vi "Top-Level.vi"() -> ()   [LabVIEW 2011]
uses:
  <vilib>/Platform/TimedLoop/XDataNode/timing_clust.ctl
  <vilib>/Platform/TimedLoop/XDataNode/nitl_modes.ctl
  <vilib>/Platform/TimedLoop/XDataNode/wakeup.ctl
  <vilib>/rvi/eio/common/nirviEmuTemplateMethod_errors.vi
  <vilib>/eio/EIONode/EIONode.xnode
  <vilib>/Platform/TimedLoop/XDataNode/XDataNode.xnode
  <vilib>/Platform/TimedLoop/XDataNode/XDNodeRunTimeDep.lvlib
panel:
  in  "manual steering":bool
  out "Velocity counts":u32
  in  "Enable AI15":bool
  out "AI15":u16 format="%04d"
  in  "Enable AI14":bool
  out "AI14":u16 format="%04d"
  in  "Enable AI13":bool
  out "AI13":u16 format="%04d"
  in  "Enable AI12":bool
  out "AI12":u16 format="%04d"
  in  "Enable AI11":bool
  out "AI11":u16 format="%04d"
  in  "Enable AI10":bool
  out "AI10":u16 format="%04d"
  in  "Enable AI9":bool
  out "AI9":u16 format="%04d"
  in  "Enable AI8":bool
  out "AI8":u16 format="%04d"
  in  "Enable AI7":bool
  out "AI7":u16 format="%04d"
  in  "Enable AI6":bool
  out "AI6":u16 format="%04d"
  in  "Enable AI5":bool
  out "AI5":u16 format="%04d"
  in  "Enable AI4":bool
  out "AI4":u16 format="%04d"
  in  "Enable AI3":bool
  out "AI3":u16 format="%04d"
  in  "Enable AI2":bool
  out "AI2":u16 format="%04d"
  in  "Enable AI1":bool=TRUE
  out "AI1":u16 format="%04d"
  in  "Enable AI0":bool=TRUE
  out "AI0":u16 format="%04d"
  in  "ADC Run":bool=TRUE
  out "ADC Channel List":u16 format="%016b"
  in  "ADC Reset":bool
  out "Steering ON 1e-7s":u32
  out "Go Duty":u8
  out "Go Frequency":u16
  out "microblaze\\xps_gpio_0_GPIO_IO_O_pin 2":i32
  in  "manual throttle":bool
  out "Brake":bool
  out "Reverse":bool
  out "Enable":bool
  in  "uBlaze Reset":bool
  out "PWM0 period (cycles)":u32=400000
  out "PWM0 duty (cycles)":u32=80000
  in  "Clock Frequency (Hz)":u32=40000000
  out "PWM1 period(cycles)":u32=400000
  out "PWM1 duty (cycles)":u32=80000
  in  "PWM0 frequency (Hz)":u16
  in  "PWM0 duty (100*%)":u16
  in  "PWM1 frequency (Hz)":u16
  in  "PWM1 duty (100*%)":u16
  out "Steering period (cycles)":u32=400000
  out "Steering duty (cycles)":u32=80000
  out "GO period (cycles)":u32=400000
  out "GO duty (cycles)":u32=80000
  in  "Steering frequency (Hz)":u16=50
  in  "Steering ON 1e-7s":u32=8
  in  "GO frequency (Hz)":u16=1000
  in  "GO duty (100*%)":u16
  # "ADC"
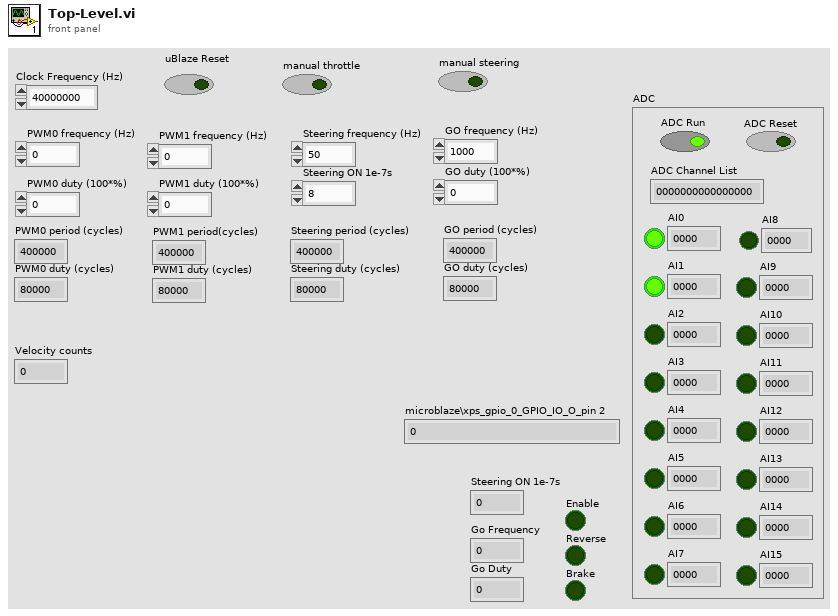
[diagram p1: front panel]
types:
  T1 = typedef "XDNodeRunTimeDep.lvlib/timing_clust.ctl" = cluster{"Expected End [f-1]":u64, "Actual End [f-1]":u64, "Finished Late? [f-1]":bool, "Expected End [i-1]":u64, "Actual End [i-1]":u64, "Finished Late? [i-1]":bool, "Expected Start [i]":u64, "Actual Start [i]":u64, "Expected Start [f]":u64, "Actual Start [f]":u64, "Source Name":string, "Structure Name":string, "Period":i64, "Deadline":i64, "Offset":i64, "Start":i64, "Priority":i32, "Timeout":i32, "Mode":T2, "Wakeup Reason":T3, "Error":errorcluster, "Source Type":string, "Secondary Source Type":string, "Global End Time":u64, "Global Start Time":u64, "Frame Duration":u64, "Iteration Duration":u64, "Assigned CPU":i32, "I/O Scan Engine Mode":u32}
  T2 = typedef "XDNodeRunTimeDep.lvlib/nitl_modes.ctl" = enum32{"No Change", "Process missed periods, maintain original phase", "Discard missed periods, maintain original phase", "Process missed periods, ignore original phase", "Discard missed periods, ignore original phase"}
  T3 = typedef "XDNodeRunTimeDep.lvlib/wakeup.ctl" = enum32{"Normal", "Aborted", "Asynchronous wakeup", "Timing source error", "Timed loop error", "Timeout"}
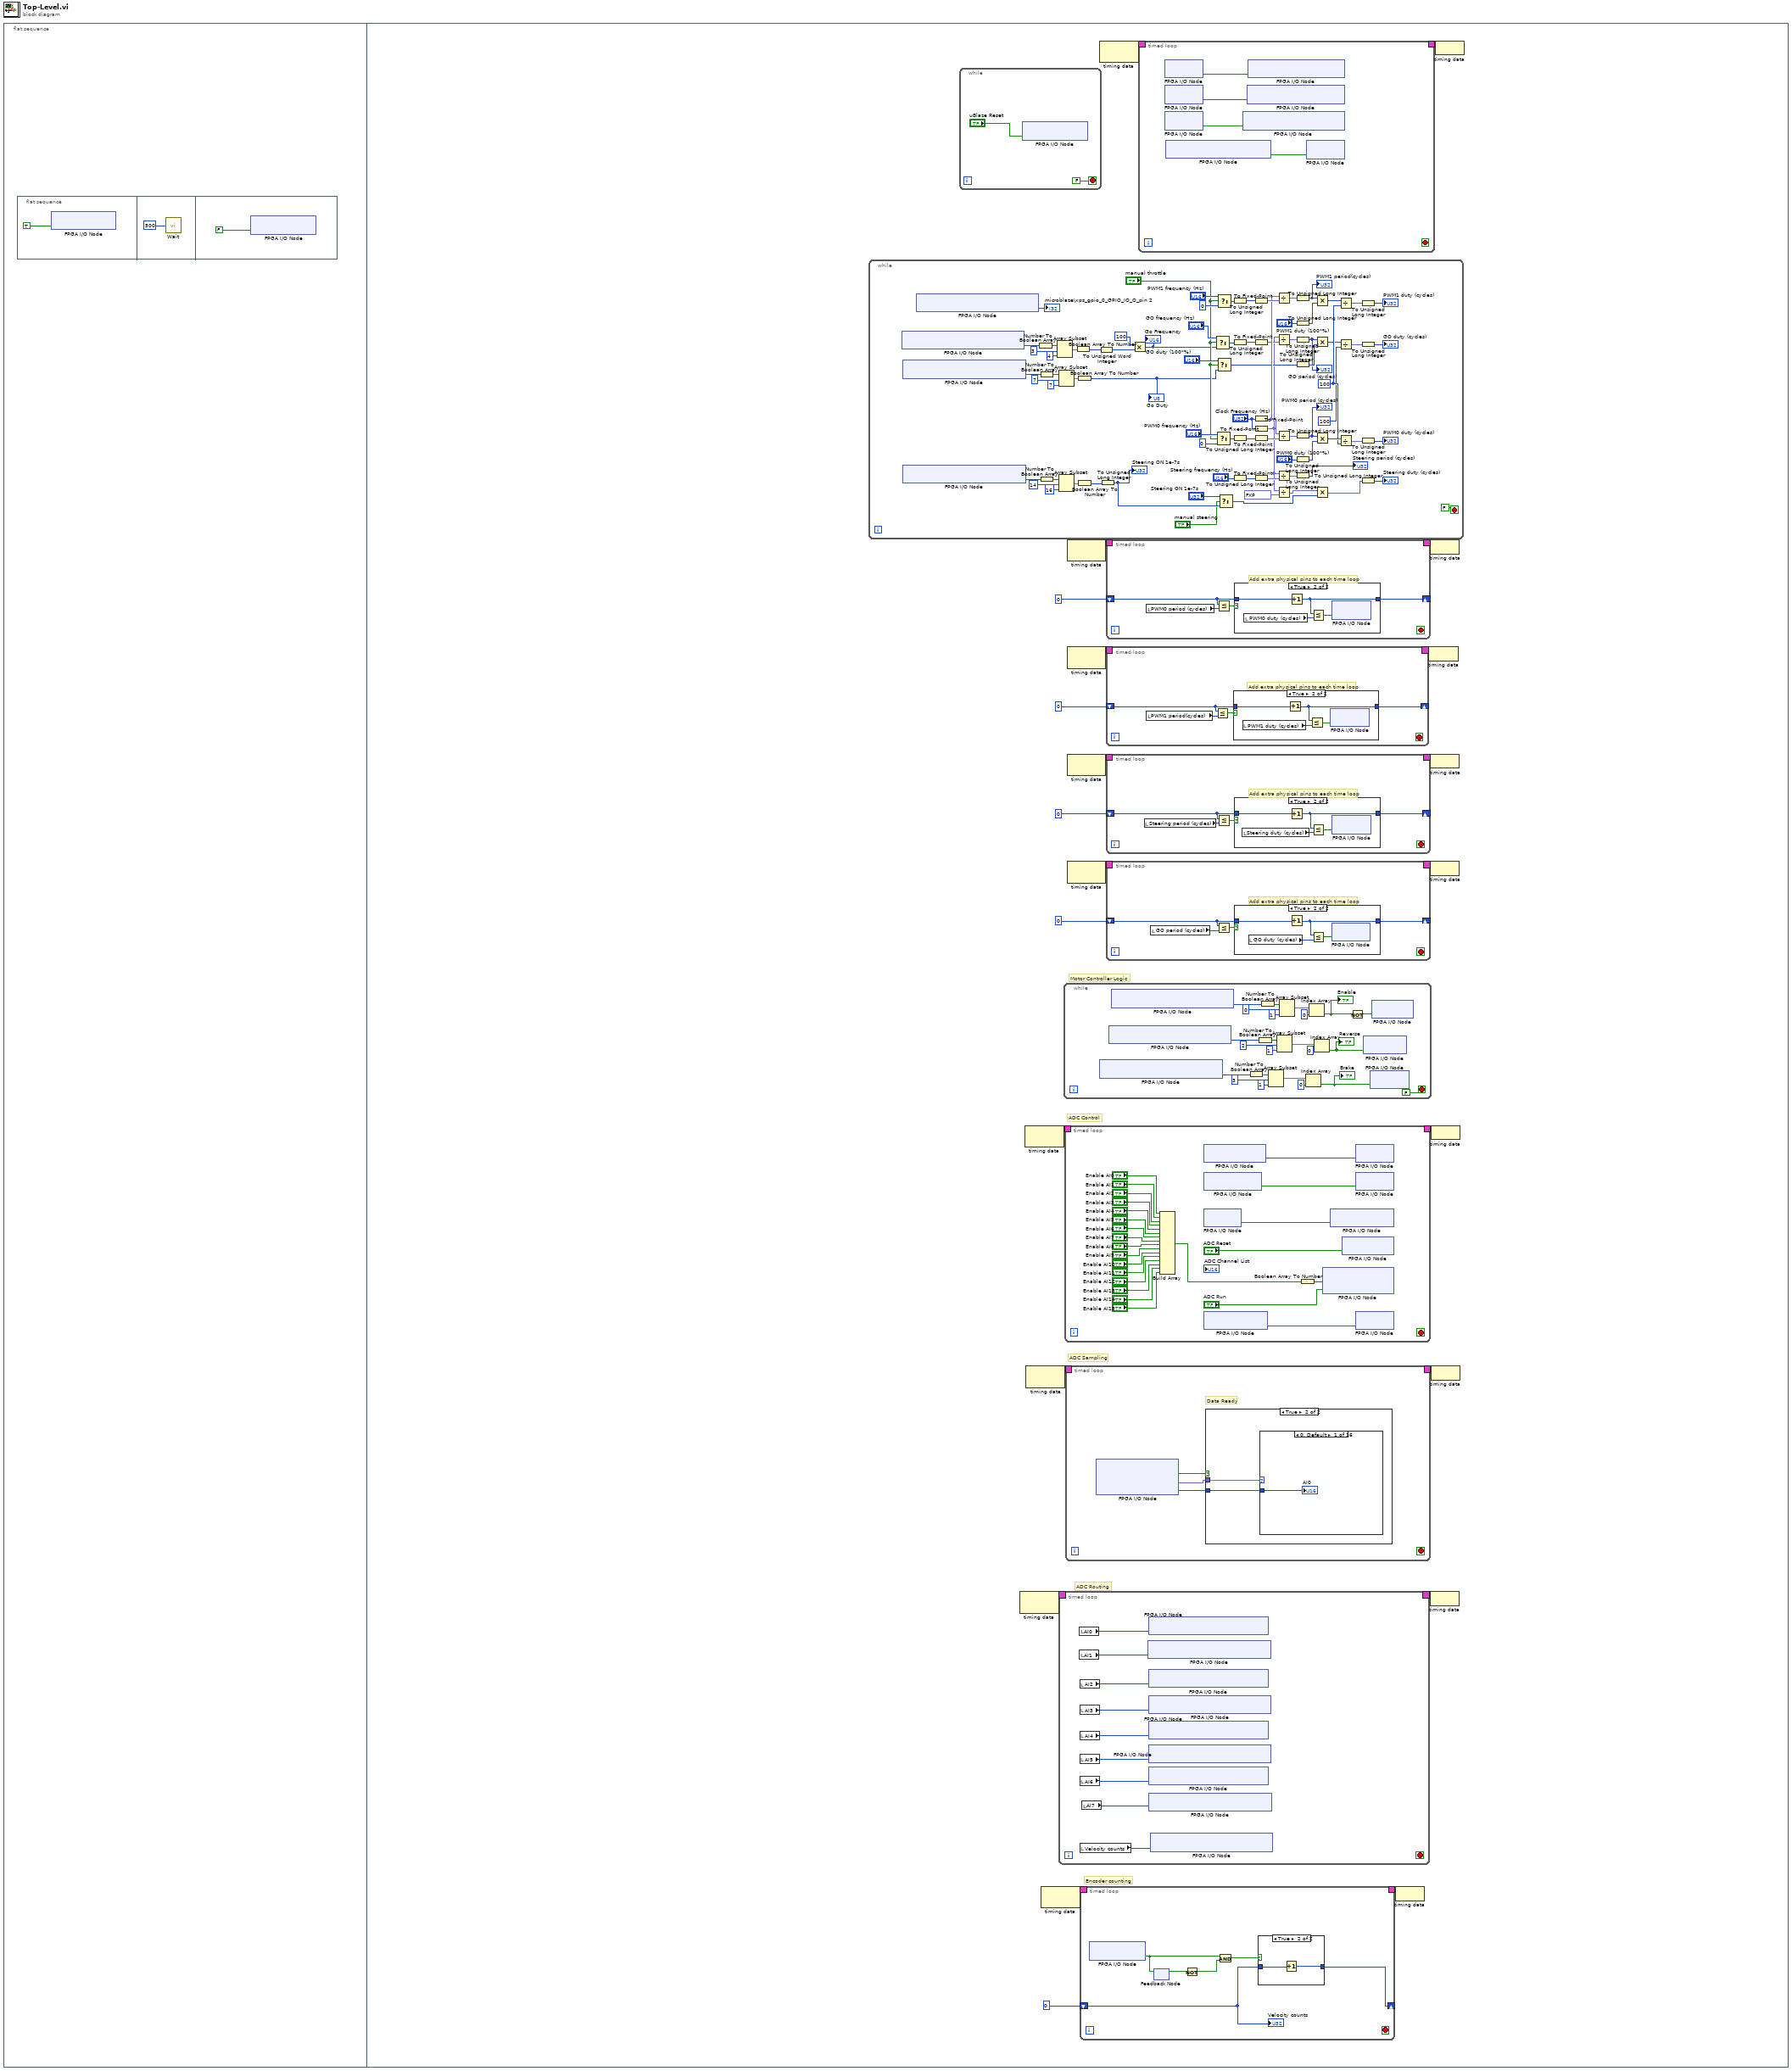
[diagram p0: block diagram]
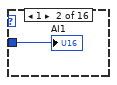
[diagram p4: hidden frame]
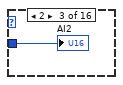
[diagram p5: hidden frame]
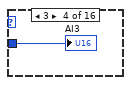
[diagram p6: hidden frame]
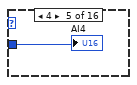
[diagram p7: hidden frame]
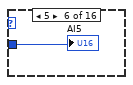
[diagram p8: hidden frame]
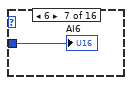
[diagram p9: hidden frame]
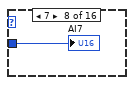
[diagram p10: hidden frame]
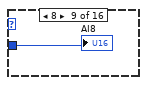
[diagram p11: hidden frame]
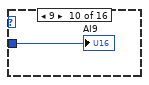
[diagram p12: hidden frame]
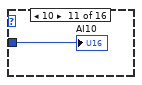
[diagram p13: hidden frame]
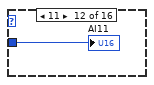
[diagram p14: hidden frame]
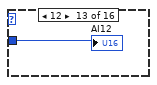
[diagram p15: hidden frame]
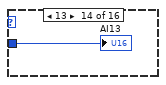
[diagram p16: hidden frame]
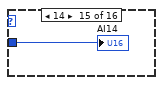
[diagram p17: hidden frame]
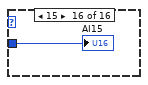
[diagram p18: hidden frame]
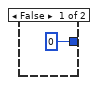
[diagram p19: hidden frame]
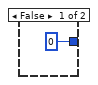
[diagram p20: hidden frame]
diagram:
  n1 = flat-sequence {
    frame #0 {
      n2 = flat-sequence {
        frame #0 {
          n3 = xnode "FPGA I/O Node"("microblaze\\reset"=TRUE ("Component-Level IP\\fpga_0_rst_1_sys_rst_pin")) -> ()  [unwired: 1 in, 1 out]
        }
        frame #1 {
          n4 = call "Wait"("Count(mSec)"=u32 500) -> ()  [unwired: 1 out]
        }
        frame #2 {
          n5 = xnode "FPGA I/O Node"("microblaze\\reset"=FALSE ("Component-Level IP\\fpga_0_rst_1_sys_rst_pin")) -> ()  [unwired: 1 in, 1 out]
        }
      }
    }
    frame #1 {
      # "Encoder counting"
      # "ADC Routing"
      # "ADC Sampling"
      # "ADC Control"
      # "Motor Controller Logic"
      n6 = while {
        stop <- FALSE stop-if-true
        w187 = u32 100 ("y")
        n7 = xnode "FPGA I/O Node"() -> ("microblaze\\xps_gpio_0_GPIO_IO_O_pin"=w152:i32)  [unwired: 1 in, 1 out]
        n8 = xnode "FPGA I/O Node"() -> ("microblaze\\xps_gpio_0_GPIO_IO_O_pin"=w146:i32)  [unwired: 1 in, 1 out]
        n9 = xnode "FPGA I/O Node"() -> ("microblaze\\xps_gpio_0_GPIO_IO_O_pin"=w147:i32)  [unwired: 1 in, 1 out]
        n10 = xnode "FPGA I/O Node"() -> ("microblaze\\xps_gpio_0_GPIO_IO_O_pin"=→"microblaze\\xps_gpio_0_GPIO_IO_O_pin 2":i32)  [unwired: 1 in, 1 out]
        n11 = Number To Boolean Array(number=w152) -> (Boolean array=w156:bool[])
        n12 = Number To Boolean Array(number=w146) -> (Boolean array=w142:bool[])
        n13 = Number To Boolean Array(number=w147) -> (Boolean array=w151:bool[])
        n14 = Array Subset(array=w156, index=3, length=4) -> (w155:bool[])
        n15 = Array Subset(array=w142, index=7, length=7) -> (w143:bool[])
        n16 = Array Subset(array=w151, index=14, length=16) -> (w150:bool[])
        n17 = Boolean Array To Number(Boolean array=w155) -> (number=w139:u8)
        n18 = Boolean Array To Number(Boolean array=w143) -> (number=w141:u8)
        "Go Duty" <- w141
        n19 = Boolean Array To Number(Boolean array=w150) -> (number=w131:u16)
        n20 = To Unsigned Word Integer(number=w139) -> (unsigned 16bit integer=w138:u16)
        n21 = To Unsigned Long Integer(number=w131) -> (unsigned 32bit integer=w130:u32)
        "Steering ON 1e-7s" <- w130
        n22 = Multiply(x=u16 100, y=w138) -> (x*y=w158:u16)
        "Go Frequency" <- w158
        n23 = Select(t="GO frequency (Hz)", s="manual throttle", f=w158) -> (s? t:f=w170:u16)
        n24 = Select(t="PWM0 frequency (Hz)", s="manual throttle", f=u16 0) -> (s? t:f=w168:u16)
        n25 = Select(t="GO duty (100*%)", s="manual throttle", f=w141) -> (s? t:f=w166:u16)
        n26 = Select(t="PWM1 frequency (Hz)", s="manual throttle", f=u16 0) -> (s? t:f=w172:u16)
        n27 = Select(t="Steering ON 1e-7s", s="manual steering", f=w130) -> (s? t:f=w133:u32)
        n28 = To Unsigned Long Integer(number=w172) -> (unsigned 32bit integer=w195:u32)
        n29 = To Unsigned Long Integer(number=w170) -> (unsigned 32bit integer=w180:u32)
        n30 = To Unsigned Long Integer(number=w168) -> (unsigned 32bit integer=w199:u32)
        n31 = To Unsigned Long Integer(number="Steering frequency (Hz)") -> (unsigned 32bit integer=w182:u32)
        n32 = To Fixed-Point(number=w195) -> (fixed-point=w194:fxp<+,32,32>)  [unwired: 1 out]
        n33 = To Fixed-Point(number=w180) -> (fixed-point=w179:fxp<+,32,32>)  [unwired: 1 out]
        n34 = To Fixed-Point(number="Clock Frequency (Hz)") -> (fixed-point=w188:fxp<+,32,32>)  [unwired: 1 out]
        n35 = To Fixed-Point(number="Clock Frequency (Hz)") -> (fixed-point=w137:fxp<+,32,32>)  [unwired: 1 out]
        n36 = To Fixed-Point(number=w199) -> (fixed-point=w200:fxp<+,32,32>)  [unwired: 1 out]
        n37 = To Fixed-Point(number=w182) -> (fixed-point=w183:fxp<+,32,32>)  [unwired: 1 out]
        n38 = Divide(x=w188, y=w194) -> (x/y=w189:fxp<+,32,33>)
        n39 = Divide(x=w137, y=w179) -> (x/y=w174:fxp<+,32,33>)
        n40 = Divide(x=w188, y=w200) -> (x/y=w205:fxp<+,32,33>)
        n41 = Divide(x=w137, y=w183) -> (x/y=w185:fxp<+,32,33>)
        n42 = Divide(x=w137, y=fxp<+,32,32> 10000000.0) -> (x/y=w134:fxp<+,64,32>)
        n43 = To Unsigned Long Integer(number=w189) -> (unsigned 32bit integer=w190:u32)
        "PWM1 period(cycles)" <- w190
        n44 = To Unsigned Long Integer(number="PWM1 duty (100*%)") -> (unsigned 32bit integer=w196:u32)
        n45 = To Unsigned Long Integer(number=w174) -> (unsigned 32bit integer=w175:u32)
        "GO period (cycles)" <- w175
        n46 = To Unsigned Long Integer(number=w166) -> (unsigned 32bit integer=w181:u32)
        n47 = To Unsigned Long Integer(number=w205) -> (unsigned 32bit integer=w204:u32)
        "PWM0 period (cycles)" <- w204
        n48 = To Unsigned Long Integer(number="PWM0 duty (100*%)") -> (unsigned 32bit integer=w197:u32)
        n49 = To Unsigned Long Integer(number=w185) -> (unsigned 32bit integer=→"Steering period (cycles)":u32)
        n50 = Multiply(x=w190, y=w196) -> (x*y=w191:u32)
        n51 = Multiply(x=w175, y=w181) -> (x*y=w176:u32)
        n52 = Multiply(x=w204, y=w197) -> (x*y=w203:u32)
        n53 = Multiply(x=w134, y=w133) -> (x*y=w132:fxp<+,64,64>)
        n54 = Divide(x=w191, y=w187) -> (x/y=w192:fxp<+,32,33>)
        n55 = Divide(x=w176, y=u32 100) -> (x/y=w177:fxp<+,32,33>)
        n56 = Divide(x=w203, y=w187) -> (x/y=w202:fxp<+,32,33>)
        n57 = To Unsigned Long Integer(number=w192) -> (unsigned 32bit integer=→"PWM1 duty (cycles)":u32)
        n58 = To Unsigned Long Integer(number=w177) -> (unsigned 32bit integer=→"GO duty (cycles)":u32)
        n59 = To Unsigned Long Integer(number=w202) -> (unsigned 32bit integer=→"PWM0 duty (cycles)":u32)
        n60 = To Unsigned Long Integer(number=w132) -> (unsigned 32bit integer=→"Steering duty (cycles)":u32)
      }
      n61 = while {
        stop <- FALSE stop-if-true
        n62 = xnode "FPGA I/O Node"("microblaze\\reset"="uBlaze Reset") -> ()  [unwired: 1 in, 1 out]
      }
      n63 = node-c288() -> (w8:T1)  [unwired: 1 in]
      n64 = node-c288() -> (w12:T1)  [unwired: 1 in]
      n65 = node-c288() -> (w10:T1)  [unwired: 1 in]
      n66 = node-c288() -> (w6:T1)  [unwired: 1 in]
      n67 = timed-loop {
        timing: w8 -> [_]
        timing-out: [_] -> w7
        stop <- _ stop-if-true
        n68 = local read "AI0"() -> (w47:u16)
        n69 = local read "AI1"() -> (w48:u16)
        n70 = local read "AI2"() -> (w46:u16)
        n71 = local read "AI3"() -> (w45:u16)
        n72 = local read "AI4"() -> (w44:u16)
        n73 = local read "AI5"() -> (w43:u16)
        n74 = local read "AI6"() -> (w42:u16)
        n75 = local read "Velocity counts"() -> (w40:u32)
        n76 = local read "AI7"() -> (w41:u16)
        n77 = xnode "FPGA I/O Node"("microblaze\\xps_gpio_1_GPIO2_IO_I_pin"=w48) -> ()  [unwired: 1 in, 1 out]
        n78 = xnode "FPGA I/O Node"("microblaze\\xps_gpio_1_GPIO_IO_I_pin"=w47) -> ()  [unwired: 1 in, 1 out]
        n79 = xnode "FPGA I/O Node"("microblaze\\xps_gpio_2_GPIO_IO_I_pin"=w46) -> ()  [unwired: 1 in, 1 out]
        n80 = xnode "FPGA I/O Node"("microblaze\\xps_gpio_2_GPIO2_IO_I_pin"=w45) -> ()  [unwired: 1 in, 1 out]
        n81 = xnode "FPGA I/O Node"("microblaze\\xps_gpio_3_GPIO_IO_I_pin"=w44) -> ()  [unwired: 1 in, 1 out]
        n82 = xnode "FPGA I/O Node"("microblaze\\xps_gpio_3_GPIO2_IO_I_pin"=w43) -> ()  [unwired: 1 in, 1 out]
        n83 = xnode "FPGA I/O Node"("microblaze\\xps_gpio_4_GPIO_IO_I_pin"=w42) -> ()  [unwired: 1 in, 1 out]
        n84 = xnode "FPGA I/O Node"("microblaze\\xps_gpio_4_GPIO2_IO_I_pin"=w41) -> ()  [unwired: 1 in, 1 out]
        n85 = xnode "FPGA I/O Node"("microblaze\\xps_gpio_5_GPIO2_IO_I_pin"=w40) -> ()  [unwired: 1 in, 1 out]
      }
      n86 = while {
        stop <- FALSE stop-if-true
        n87 = xnode "FPGA I/O Node"() -> ("microblaze\\xps_gpio_0_GPIO_IO_O_pin"=w115:i32)  [unwired: 1 in, 1 out]
        n88 = xnode "FPGA I/O Node"() -> ("microblaze\\xps_gpio_0_GPIO_IO_O_pin"=w122:i32)  [unwired: 1 in, 1 out]
        n89 = xnode "FPGA I/O Node"() -> ("microblaze\\xps_gpio_0_GPIO_IO_O_pin"=w125:i32)  [unwired: 1 in, 1 out]
        n90 = Number To Boolean Array(number=w115) -> (Boolean array=w118:bool[])
        n91 = Number To Boolean Array(number=w122) -> (Boolean array=w119:bool[])
        n92 = Number To Boolean Array(number=w125) -> (Boolean array=w128:bool[])
        n93 = Array Subset(array=w118, index=3, length=1) -> (w112:bool[])
        n94 = Array Subset(array=w119, index=2, length=1) -> (w113:bool[])
        n95 = Array Subset(array=w128, index=0, length=1) -> (w109:bool[])
        n96 = Index Array(array=w112, index=0) -> (element=w110:bool)
        "Brake" <- w110
        n97 = Index Array(array=w109, index=0) -> (element=w107:bool)
        "Enable" <- w107
        n98 = Index Array(array=w113, index=0) -> (element=w111:bool)
        "Reverse" <- w111
        n99 = Not(x=w107) -> (.not. x?=w108:bool)
        n100 = xnode "FPGA I/O Node"("REVERSE"=w111) -> ()  [unwired: 1 in, 1 out]
        n101 = xnode "FPGA I/O Node"("BRAKE"=w110) -> ()  [unwired: 1 in, 1 out]
        n102 = xnode "FPGA I/O Node"("ENABLE"=w108) -> ()  [unwired: 1 in, 1 out]
      }
      n103 = timed-loop {
        timing: w12 -> [_]
        timing-out: [_] -> w11
        stop <- _ stop-if-true
        n104 = Build Array("Enable AI0", "Enable AI1", "Enable AI2", "Enable AI3", "Enable AI4", "Enable AI5", "Enable AI6", "Enable AI7", "Enable AI8", "Enable AI9", "Enable AI10", "Enable AI11", "Enable AI12", "Enable AI13", "Enable AI14", "Enable AI15") -> (w94:bool[])
        n105 = xnode "FPGA I/O Node"() -> ("ADC\\aaispics_n"=w96:bool)  [unwired: 1 in, 1 out]
        n106 = xnode "FPGA I/O Node"() -> ("ADC\\aaispiclk"=w97:bool)  [unwired: 1 in, 1 out]
        n107 = xnode "FPGA I/O Node"() -> ("SDO"=w98:bool)  [unwired: 1 in, 1 out]
        n108 = xnode "FPGA I/O Node"() -> ("ADC\\aaispimosi"=w99:bool)  [unwired: 1 in, 1 out]
        n109 = Boolean Array To Number(Boolean array=w94) -> (number=w95:u16)
        n110 = xnode "FPGA I/O Node"("ADC\\caichannellist"=w95, "ADC\\cairun"="ADC Run") -> ()  [unwired: 2 in, 2 out]
        n111 = xnode "FPGA I/O Node"("ADC\\aaispimiso"=w98) -> ()  [unwired: 1 in, 1 out]
        n112 = xnode "FPGA I/O Node"("ADC\\areset"="ADC Reset") -> ()  [unwired: 1 in, 1 out]
        n113 = xnode "FPGA I/O Node"("CS"=w96) -> ()  [unwired: 1 in, 1 out]
        n114 = xnode "FPGA I/O Node"("SCLK"=w97) -> ()  [unwired: 1 in, 1 out]
        n115 = xnode "FPGA I/O Node"("SDI"=w99) -> ()  [unwired: 1 in, 1 out]
      }
      n116 = timed-loop {
        timing: w10 -> [_]
        timing-out: [_] -> w9
        stop <- _ stop-if-true
        # "Data Ready"
        n117 = xnode "FPGA I/O Node"() -> ("ADC\\caidataready"=w55:bool, "ADC\\caicurrentchannel"=w53:fxp<+,4,4>, "ADC\\caidataout"=w54:u16)  [unwired: 3 in, 3 out]
        n118 = case shown="True" w55 {
          tunnel: w53 -> [_ w57]
          tunnel: w54 -> [_ w56]
          frame False {
          }
          frame True {
            n119 = case shown="0, Default" w57 {
              tunnel: w56 -> [w58 w59 w60 w61 w62 w63 w64 w65 w66 w67 w68 w69 w70 w71 w72 w73]
              frame 0, Default {
                "AI0" <- w58
              }
              frame 1 {
                "AI1" <- w59
              }
              frame 2 {
                "AI2" <- w60
              }
              frame 3 {
                "AI3" <- w61
              }
              frame 4 {
                "AI4" <- w62
              }
              frame 5 {
                "AI5" <- w63
              }
              frame 6 {
                "AI6" <- w64
              }
              frame 7 {
                "AI7" <- w65
              }
              frame 8 {
                "AI8" <- w66
              }
              frame 9 {
                "AI9" <- w67
              }
              frame 10 {
                "AI10" <- w68
              }
              frame 11 {
                "AI11" <- w69
              }
              frame 12 {
                "AI12" <- w70
              }
              frame 13 {
                "AI13" <- w71
              }
              frame 14 {
                "AI14" <- w72
              }
              frame 15 {
                "AI15" <- w73
              }
            }
          }
        }
      }
      n120 = node-c288() -> (w24:T1)  [unwired: 1 out]
      n121 = node-c288() -> (w22:T1)  [unwired: 1 out]
      n122 = node-c288() -> (w20:T1)  [unwired: 1 out]
      n123 = node-c288() -> (w18:T1)  [unwired: 1 out]
      n124 = timed-loop {
        timing: w6 -> [_]
        timing-out: [_] -> w5
        shift-right: [w28] -> _
        shift-left: u32 0 -> [w27]
        stop <- _ stop-if-true
        n125 = xnode "FPGA I/O Node"() -> ("ENCODER_IN"=w30:bool)  [unwired: 1 in, 1 out]
        n126 = feedback-in #1(w30) -> ()
        n127 = feedback #1() -> (w31:bool)  [unwired: 1 in]
        n128 = Not(x=w31) -> (.not. x?=w32:bool)
        n129 = And(x=w30, y=w32) -> (x .and. y?=w29:bool)
        n130 = case shown="True" w29 {
          tunnel: w27 -> [w33 w35]
          tunnel: [w33 w34] -> w28
          frame False {
          }
          frame True {
            n131 = Increment(x=w35) -> (x+1=w34:u32)
          }
        }
        "Velocity counts" <- w27
      }
      n132 = node-c288() -> (w26:T1)  [unwired: 1 in]
      n133 = timed-loop {
        timing: w24 -> [_]
        timing-out: [_] -> w23
        shift-right: [w249] -> _
        shift-left: u32 0 -> [w250]
        stop <- _ stop-if-true
        # "Add extra physical pins to each time loop"
        n134 = local read "PWM0 period (cycles)"() -> (w248:u32)
        n135 = Less Or Equal?(x=w250, y=w248) -> (x <= y?=w251:bool)
        n136 = case shown="True" w251 {
          tunnel: w250 -> [_ w256]
          tunnel: [i16 0 w255] -> w249
          frame False {
          }
          frame True {
            n137 = local read "PWM0 duty (cycles)"() -> (w254:u32)
            n138 = Increment(x=w256) -> (x+1=w255:u32)
            n139 = Less Or Equal?(x=w255, y=w254) -> (x <= y?=w253:bool)
            n140 = xnode "FPGA I/O Node"("PWM0"=w253) -> ()  [unwired: 1 in, 1 out]
          }
        }
      }
      n141 = timed-loop {
        timing: w22 -> [_]
        timing-out: [_] -> w21
        shift-right: [w236] -> _
        shift-left: u32 0 -> [w237]
        stop <- _ stop-if-true
        # "Add extra physical pins to each time loop"
        n142 = local read "PWM1 period(cycles)"() -> (w235:u32)
        n143 = Less Or Equal?(x=w237, y=w235) -> (x <= y?=w238:bool)
        n144 = case shown="True" w238 {
          tunnel: w237 -> [_ w243]
          tunnel: [i16 0 w242] -> w236
          frame False {
          }
          frame True {
            n145 = local read "PWM1 duty (cycles)"() -> (w241:u32)
            n146 = Increment(x=w243) -> (x+1=w242:u32)
            n147 = Less Or Equal?(x=w242, y=w241) -> (x <= y?=w240:bool)
            n148 = xnode "FPGA I/O Node"("PWM1"=w240) -> ()  [unwired: 1 in, 1 out]
          }
        }
      }
      n149 = timed-loop {
        timing: w20 -> [_]
        timing-out: [_] -> w19
        shift-right: [w223] -> _
        shift-left: u32 0 -> [w224]
        stop <- _ stop-if-true
        # "Add extra physical pins to each time loop"
        n150 = local read "Steering period (cycles)"() -> (w222:u32)
        n151 = Less Or Equal?(x=w224, y=w222) -> (x <= y?=w225:bool)
        n152 = case shown="True" w225 {
          tunnel: w224 -> [_ w230]
          tunnel: [i16 0 w229] -> w223
          frame False {
          }
          frame True {
            n153 = local read "Steering duty (cycles)"() -> (w228:u32)
            n154 = Increment(x=w230) -> (x+1=w229:u32)
            n155 = Less Or Equal?(x=w229, y=w228) -> (x <= y?=w227:bool)
            n156 = xnode "FPGA I/O Node"("PWM2"=w227) -> ()  [unwired: 1 in, 1 out]
          }
        }
      }
      n157 = timed-loop {
        timing: w18 -> [_]
        timing-out: [_] -> w17
        shift-right: [w210] -> _
        shift-left: u32 0 -> [w211]
        stop <- _ stop-if-true
        # "Add extra physical pins to each time loop"
        n158 = local read "GO period (cycles)"() -> (w209:u32)
        n159 = Less Or Equal?(x=w211, y=w209) -> (x <= y?=w212:bool)
        n160 = case shown="True" w212 {
          tunnel: w211 -> [_ w217]
          tunnel: [i16 0 w216] -> w210
          frame False {
          }
          frame True {
            n161 = local read "GO duty (cycles)"() -> (w215:u32)
            n162 = Increment(x=w217) -> (x+1=w216:u32)
            n163 = Less Or Equal?(x=w216, y=w215) -> (x <= y?=w214:bool)
            n164 = xnode "FPGA I/O Node"("GO"=w214) -> ()  [unwired: 1 in, 1 out]
          }
        }
      }
      n165 = timed-loop {
        timing: w26 -> [_]
        timing-out: [_] -> w25
        stop <- _ stop-if-true
        n166 = xnode "FPGA I/O Node"() -> ("TCK"=w264:bool)  [unwired: 1 in, 1 out]
        n167 = xnode "FPGA I/O Node"() -> ("TMS"=w263:bool)  [unwired: 1 in, 1 out]
        n168 = xnode "FPGA I/O Node"() -> ("TDI"=w262:bool)  [unwired: 1 in, 1 out]
        n169 = xnode "FPGA I/O Node"() -> ("microblaze\\mdm_0_extTDO_pin"=w261:bool)  [unwired: 1 in, 1 out]
        n170 = xnode "FPGA I/O Node"("microblaze\\mdm_0_extTDI_pin"=w262) -> ()  [unwired: 1 in, 1 out]
        n171 = xnode "FPGA I/O Node"("microblaze\\mdm_0_TMS_pin"=w263) -> ()  [unwired: 1 in, 1 out]
        n172 = xnode "FPGA I/O Node"("microblaze\\mdm_0_TCK_pin"=w264) -> ()  [unwired: 1 in, 1 out]
        n173 = xnode "FPGA I/O Node"("TDO"=w261) -> ()  [unwired: 1 in, 1 out]
      }
      n174 = node-c288(w5) -> ()
      n175 = node-c288(w21) -> ()
      n176 = node-c288(w7) -> ()
      n177 = node-c288(w23) -> ()
      n178 = node-c288(w19) -> ()
      n179 = node-c288(w17) -> ()
      n180 = node-c288(w11) -> ()
      n181 = node-c288(w9) -> ()
      n182 = node-c288(w25) -> ()
    }
  }
